vi "Test.vi"() -> ()   [LabVIEW 2026]
uses:
  User32.dll
panel:
  out "return type 3":i16
  out "return type":i16
  out "vKey":i16
  out "return type 2":i16
  in  "y position":i32=200
  in  "x position":i32=200
  in  "Stop":bool
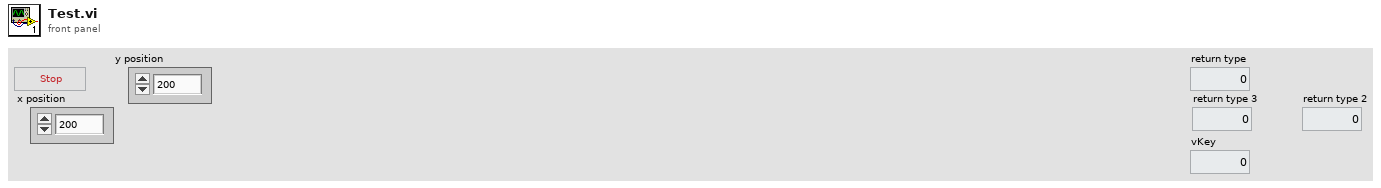
[diagram p1: front panel]
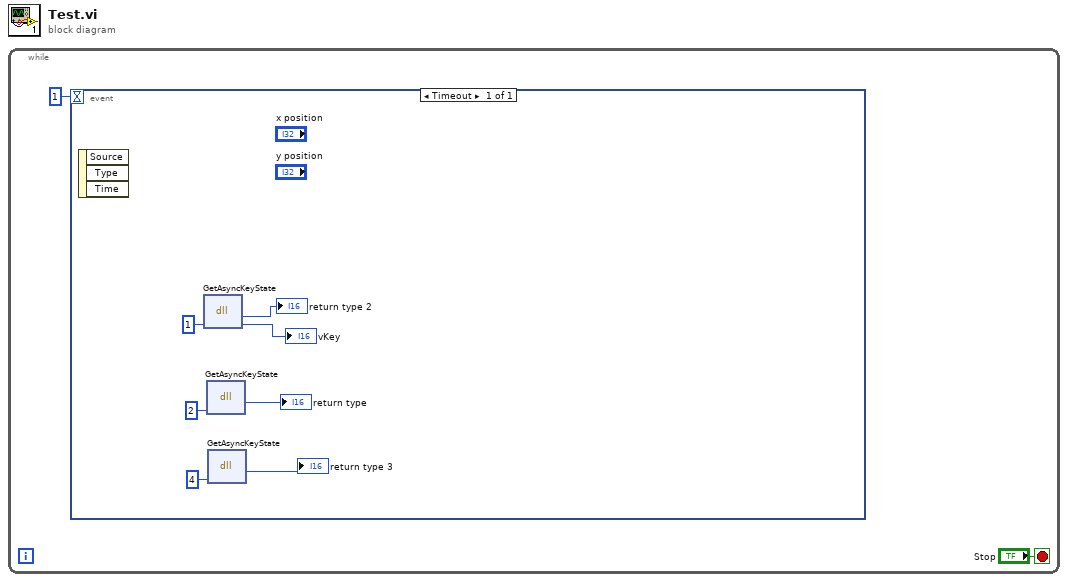
[diagram p0: block diagram]
diagram:
  n1 = while {
    stop <- "Stop" stop-if-true
    n2 = event shown="[0] Timeout" {
      selector: _ -> [_]
      dyn-events: _ -> [_]
      timeout: 1 -> [_]
      event Timeout {
        n3 = event-data() -> ()  [unwired: 1 in, 3 out]
        n4 = dll-call lib="User32.dll" fn="GetAsyncKeyState" label="Left Button Click"("vKey"=i16 1) -> ("return type"=→"return type 2":i16, "vKey"=→"vKey":i16)  [unwired: 3 in, 2 out]
        n5 = dll-call lib="User32.dll" fn="GetAsyncKeyState" label="Right Button Click"("vKey"=i16 2) -> ("return type"=→"return type":i16)  [unwired: 4 in, 2 out]
        n6 = dll-call lib="User32.dll" fn="GetAsyncKeyState" label="Middle Button Click"("vKey"=i16 4) -> ("return type"=→"return type 3":i16)  [unwired: 4 in, 2 out]
      }
    }
  }
